vi "G#Object_IsCallToParent.vi"(5 "error in (no error)":errorcluster) -> (15 "is call to parent method?":bool, 19 "error out":errorcluster)   [LabVIEW 2017, in "G#Object.lvclass"]
doc: "Checks if the caller of this VI is made as a \"Call parent method\"."
uses:
  <vilib>/addons/_AddQ/G#Object/G#Object.lvclass
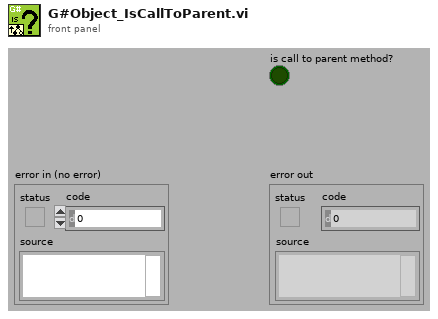
[diagram p1: front panel]
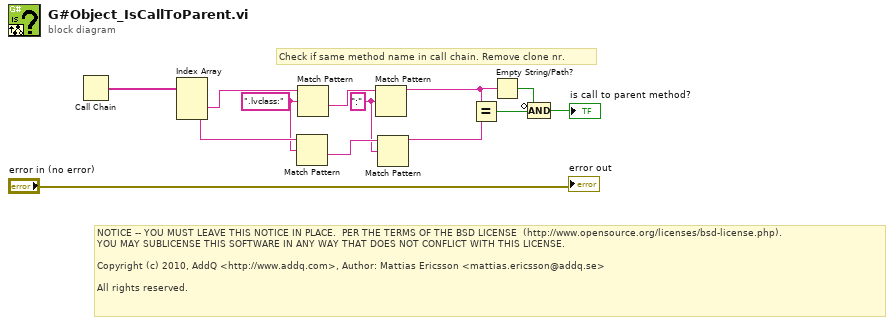
[diagram p0: block diagram]
diagram:
  w7 = ":" ("regular expression")
  w6 = ".lvclass:" ("regular expression")
  # "NOTICE -- YOU MUST LEAVE THIS NOTICE IN PLACE.  PER THE TERMS OF THE BSD LICENSE  (http://www.opensource.org/licenses/bsd-license.php).\nYOU MAY SUBLICENSE THIS SOFTWARE IN ANY WAY THAT DOES NOT CONFLICT WITH THIS LICENSE.\n\nCopyright (c) 2010, AddQ <http://www.addq.com>, Author: Mattias Ericsson <mattias.ericsson@addq.se>\n\nAll rights reserved."
  # "Check if same method name in call chain. Remove clone nr."
  n1 = Call Chain() -> (call chain=w5:string[])
  n2 = Index Array(array=w5) -> (element #2=w11:string, element #3=w12:string)  [unwired: 3 in, 1 out]
  n3 = Match Pattern(string=w12, regular expression=w6) -> (after substring=w9:string)  [unwired: 1 in, 3 out]
  n4 = Match Pattern(string=w11, regular expression=w6) -> (after substring=w10:string)  [unwired: 1 in, 3 out]
  n5 = Match Pattern(string=w10, regular expression=w7) -> (before substring=w4:string)  [unwired: 1 in, 3 out]
  n6 = Match Pattern(string=w9, regular expression=w7) -> (before substring=w8:string)  [unwired: 1 in, 3 out]
  n7 = Equal?(x=w4, y=w8) -> (x = y?=w3:bool)
  n8 = Empty String/Path?(string/path=w4) -> (empty?=w2:bool)
  n9 = Compound Arithmetic op=AND(invert w2, w3) -> (→"is call to parent method?":bool)
  "error out" <- "error in (no error)"
